vi "Get WT Data.vi"(2 "Device Info":T1) -> (0 "Error out":errorcluster)   [LabVIEW 2022 SP3]
uses:
  Anemometry/Anemometry Sub Vis/Acquisition/Device ID port info.ctl
  Anemometry/Anemometry Sub Vis/Acquisition/Sub_vis/Upload Data.ctl
  Anemometry/Anemometry Sub Vis/Globals/Meas_global.vi
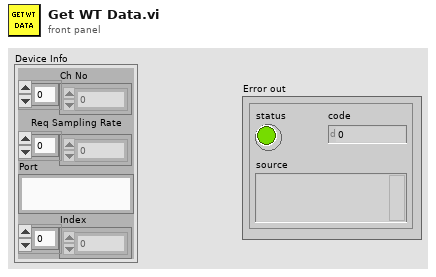
[diagram p1: front panel]
types:
  T1 = typedef "Device ID port info.ctl" = cluster{"Ch No":i16[], "Req Sampling Rate":dbl[], "Port":string, "Index":i32[]}
  T2 = typedef "Upload Data.ctl" = enum16{"Voltage Array", "Time Trace Cluster"}
  T3 = typedef "CTRL_Data_Out.ctl" = cluster{"RPM (/min)":sgl, "I_motor (A)":sgl, "V_photo (V)":sgl, "Duty (-1...1)":sgl}
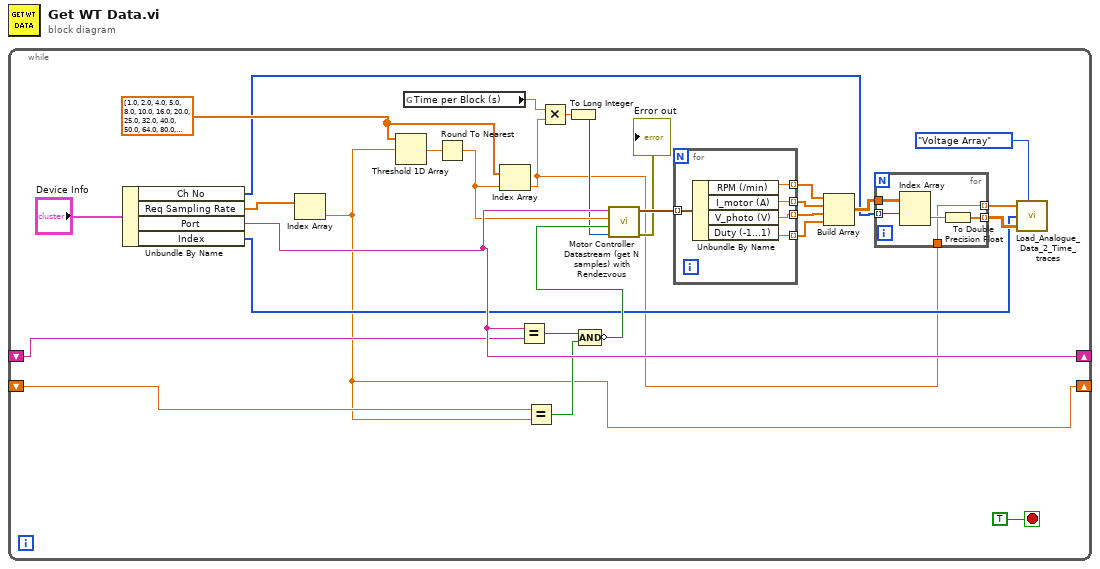
[diagram p0: block diagram]
diagram:
  n1 = while {
    shift-right: [w27] -> _
    shift-left: _ -> [w26]
    shift-right: [w1] -> _
    shift-left: _ -> [w25]
    stop <- TRUE stop-if-true
    w18 = dbl[] [1.0, 2.0, 4.0, 5.0, 8.0, 10.0, 16.0, 20.0, 25.0, 32.0, 40.0, 50.0, 64.0, 80.0, 100.0, 125.0, 160.0, 200.0, 250.0, 320.0, 400.0, 500.0, 625.0, 800.0] ("Array")
    n2 = Unbundle By Name("Device Info") -> ("Ch No"=w5:i16[], "Req Sampling Rate"=w28:dbl[], "Port"=w27:string, "Index"=w4:i32[])
    n3 = Index Array(array=w28) -> (element=w1:dbl)  [unwired: 1 in]
    n4 = Threshold 1D Array(2:w1, 3:w18) -> (0:w21:dbl)  [unwired: 1 in]
    n5 = global read "Meas_global.vi" "Time per Block (s)"() -> (w19:dbl)
    n6 = Round To Nearest(number=w21) -> (nearest integer value=w17:dbl)
    n7 = Index Array(array=w18, index=w17) -> (element=w2:dbl)
    n8 = Equal?(x=w27, y=w26) -> (x = y?=w24:bool)
    n9 = Equal?(x=w25, y=w1) -> (x = y?=w23:bool)
    n10 = Multiply(x=w19, y=w2) -> (x*y=w20:dbl)
    n11 = To Long Integer(number=w20) -> (32bit integer=w16:i32)
    n12 = Compound Arithmetic op=AND(w24, w23) -> (invert w22:bool)
    n13 = call "Motor Controller Datastream (get N samples) with Rendezvous.vi"("N samples"=w16, "Set data rate?"=w22, "Data rate (Hz)"=w17, "COM port"=w27) -> ("Error out"=→"Error out":errorcluster, "Data cluster array"=w15:T3[])  [unwired: 4 in, 2 out]
    n14 = for {
      tunnel: w15 -> [w39] mode=indexing
      tunnel: [w38] -> w13 mode=indexing
      tunnel: [w37] -> w12 mode=indexing
      tunnel: [w36] -> w11 mode=indexing
      tunnel: [w35] -> w10 mode=indexing
      n15 = Unbundle By Name(w39) -> ("RPM (/min)"=w35:sgl, "I_motor (A)"=w36:sgl, "V_photo (V)"=w37:sgl, "Duty (-1...1)"=w38:sgl)
    }
    n16 = Build Array(w10, w11, w12, w13) -> (w6:sgl[][])
    n17 = for {
      tunnel: w5 -> [w33] mode=indexing
      tunnel: w6 -> [w34]
      tunnel: w2 -> [w30]
      tunnel: [w31] -> w8 mode=indexing
      tunnel: [w30] -> w7 mode=indexing
      n18 = Index Array(array=w34, index (row)=w33) -> (element=w32:sgl[])  [unwired: 1 in]
      n19 = To Double Precision Float(number=w32) -> (double precision float=w31:dbl[])
    }
    n20 = call "Load_Analogue_Data_2_Time_traces.vi"("Sampling Rate (Hz)"=w7, "Mode"=Upload_Data."Voltage Array", "Index"=w4, "Voltage Array"=w8) -> ()  [unwired: 3 in]
  }
